vi "AbortSystemConfiguration.vi"(0 "File Path":path) -> ()   [LabVIEW 2021]
uses:
  <vilib>/Utility/file.llb/Write Delimited Spreadsheet (string).vi
  <vilib>/Utility/file.llb/Write Delimited Spreadsheet (I64).vi
  <vilib>/Utility/file.llb/Write Delimited Spreadsheet (DBL).vi
panel:
  in  "?":bool
  in  "?":bool
  out "Row":i32[](array[numeric])
  in  "Row":i32
  in  "Remove Event":bool
  in  "Add Event":bool
  in  "Sensor Select":u16(ring) items=["", "PT1", "PT2", "PT3", "TC1", "TC2", "LP1", "VS", "VLJ", "VR", "N2O Flowrate", "Ethanol Flowrate"]
  in  "Low Threshold":dbl
  in  "High Threshold":dbl
  in  "P#":i32
  in  "Event Name":string
  in  "SV6":bool
  in  "SV5":bool
  out "?":bool[](array[boolean])
  out "?":bool[](array[boolean])
  in  "SV4":bool
  out "?":bool[](array[boolean])
  in  "SV3":bool
  in  "SV2":bool
  in  "SV1":bool
  out "?":bool[](array[boolean])
  out "?":bool[](array[boolean])
  out "?":bool[](array[boolean])
  in  "SV0":bool
  out "?":dbl[](array[numeric])
  out "?":u16[](array[ring]) items=["", "PT1", "PT2", "PT3", "TC1", "TC2", "LP1", "VS", "VLJ", "VR", "N2O FLowrate", "Ethanol Flowrate"]
  out "?":string[](array[string])
  out "?":bool[](array[boolean])
  out "?":i32[](array[numeric])
  out "?":dbl[](array[numeric])
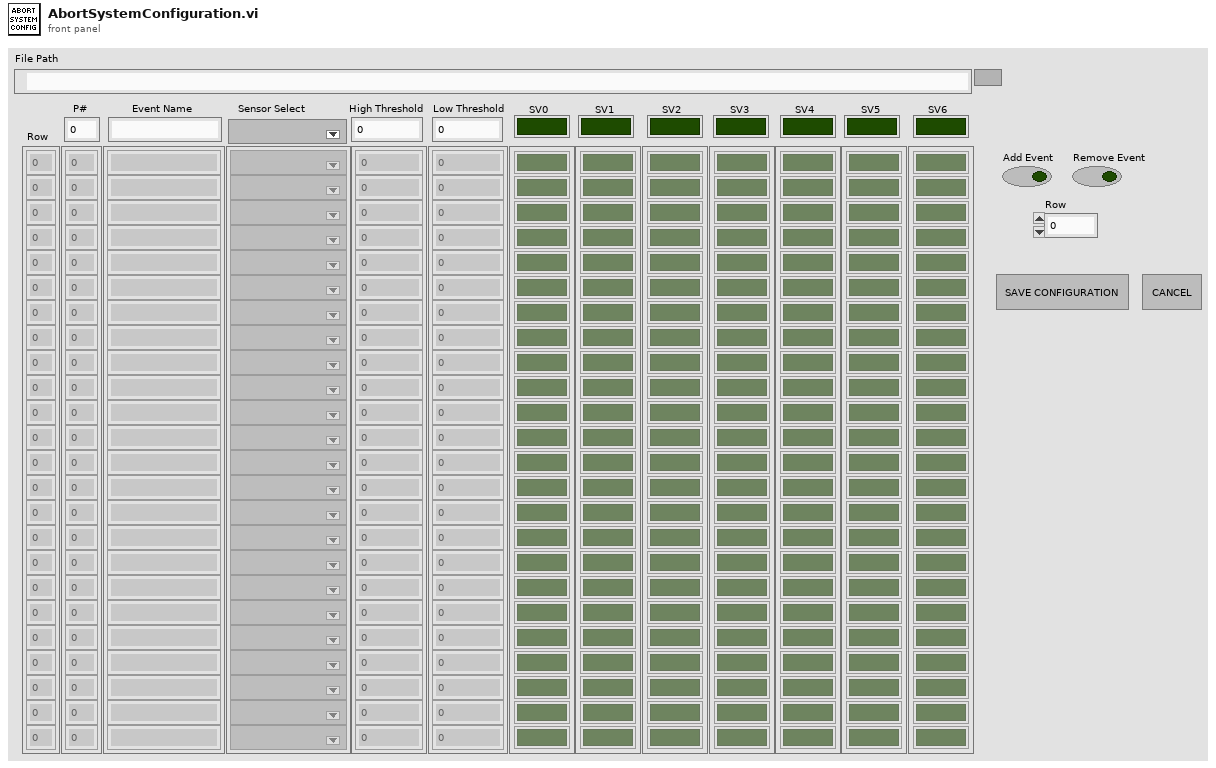
[diagram p1: front panel]
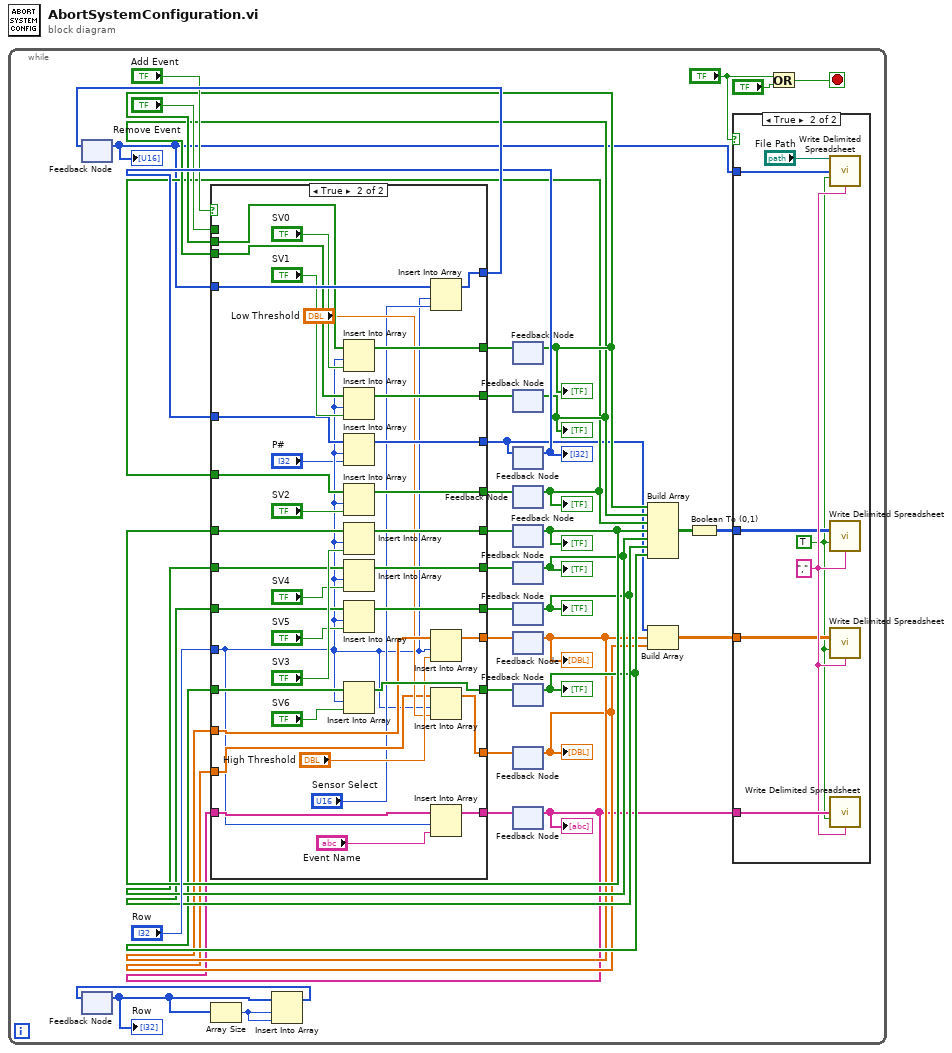
[diagram p0: block diagram]
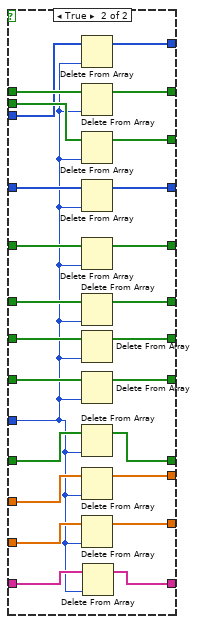
[diagram p4: hidden frame]
diagram:
  n1 = while {
    stop <- w3 stop-if-true
    n2 = feedback #1() -> (w5:u16[])  [unwired: 1 in]
    "?" <- w5
    n3 = feedback #2() -> (w22:i32[])  [unwired: 1 in]
    "Row" <- w22
    n4 = Array Size(array=w22) -> (size(s)=w21:i32)
    n5 = Insert Into Array(array=w22, index=w21, new element=w21) -> (w23:i32[])
    n6 = feedback-in #2(w23) -> ()
    n7 = feedback #3() -> (w18:bool[])  [unwired: 1 in]
    "?" <- w18
    n8 = feedback #4() -> (w17:bool[])  [unwired: 1 in]
    "?" <- w17
    n9 = feedback #5() -> (w27:i32[])  [unwired: 1 in]
    "?" <- w27
    n10 = feedback #6() -> (w16:bool[])  [unwired: 1 in]
    "?" <- w16
    n11 = feedback #7() -> (w15:bool[])  [unwired: 1 in]
    "?" <- w15
    n12 = feedback #8() -> (w14:bool[])  [unwired: 1 in]
    "?" <- w14
    n13 = feedback #9() -> (w13:bool[])  [unwired: 1 in]
    "?" <- w13
    n14 = feedback #10() -> (w11:dbl[])  [unwired: 1 in]
    "?" <- w11
    n15 = feedback #11() -> (w12:bool[])  [unwired: 1 in]
    "?" <- w12
    n16 = feedback #12() -> (w10:dbl[])  [unwired: 1 in]
    "?" <- w10
    n17 = feedback #13() -> (w8:string[])  [unwired: 1 in]
    "?" <- w8
    n18 = case shown="True" "Add Event" {
      tunnel: "Row" -> [w44 w108]
      tunnel: [w57 w143] -> w36
      tunnel: w5 -> [w56 w142]
      tunnel: [w63 w139] -> w35
      tunnel: w18 -> [w62 w138]
      tunnel: [w60 w137] -> w34
      tunnel: w17 -> [w61 w136]
      tunnel: [w69 w134] -> w33
      tunnel: w16 -> [w68 w133]
      tunnel: w15 -> [w66 w131]
      tunnel: [w67 w130] -> w32
      tunnel: w14 -> [w64 w128]
      tunnel: [w65 w127] -> w31
      tunnel: w13 -> [w58 w125]
      tunnel: [w59 w124] -> w30
      tunnel: w12 -> [w55 w123]
      tunnel: [w54 w122] -> w29
      tunnel: w8 -> [w52 w120]
      tunnel: [w53 w119] -> w28
      tunnel: w27 -> [w50 w117]
      tunnel: [w51 w116] -> w9
      tunnel: w11 -> [w46 w114]
      tunnel: [w47 w113] -> w26
      tunnel: w10 -> [w48 w111]
      tunnel: [w49 w110] -> w25
      tunnel: "Remove Event" -> [w45 _]
      frame False {
        n19 = case shown="False" w45 {
          tunnel: [w70 w106] -> w69
          tunnel: w68 -> [w70 w105]
          tunnel: [w72 w104] -> w67
          tunnel: w66 -> [w72 w103]
          tunnel: [w73 w102] -> w65
          tunnel: w64 -> [w73 w101]
          tunnel: [w74 w100] -> w63
          tunnel: w62 -> [w74 w99]
          tunnel: w61 -> [w76 w98]
          tunnel: [w76 w97] -> w60
          tunnel: [w77 w96] -> w59
          tunnel: w58 -> [w77 w95]
          tunnel: [w71 w94] -> w57
          tunnel: w56 -> [w71 w93]
          tunnel: w55 -> [w81 w92]
          tunnel: [w81 w91] -> w54
          tunnel: [w80 w90] -> w53
          tunnel: w52 -> [w80 w89]
          tunnel: [w79 w88] -> w51
          tunnel: w50 -> [w79 w87]
          tunnel: [w78 w86] -> w49
          tunnel: w48 -> [w78 w85]
          tunnel: [w75 w84] -> w47
          tunnel: w46 -> [w75 w83]
          tunnel: w44 -> [_ w82]
          frame False {
          }
          frame True {
            n20 = Delete From Array(array=w93, index=w82) -> (array with subset deleted=w94:u16[])  [unwired: 1 in, 1 out]
            n21 = Delete From Array(array=w99, index=w82) -> (array with subset deleted=w100:bool[])  [unwired: 1 in, 1 out]
            n22 = Delete From Array(array=w98, index=w82) -> (array with subset deleted=w97:bool[])  [unwired: 1 in, 1 out]
            n23 = Delete From Array(array=w87, index=w82) -> (array with subset deleted=w88:i32[])  [unwired: 1 in, 1 out]
            n24 = Delete From Array(array=w105, index=w82) -> (array with subset deleted=w106:bool[])  [unwired: 1 in, 1 out]
            n25 = Delete From Array(array=w103, index=w82) -> (array with subset deleted=w104:bool[])  [unwired: 1 in, 1 out]
            n26 = Delete From Array(array=w101, index=w82) -> (array with subset deleted=w102:bool[])  [unwired: 1 in, 1 out]
            n27 = Delete From Array(array=w95, index=w82) -> (array with subset deleted=w96:bool[])  [unwired: 1 in, 1 out]
            n28 = Delete From Array(array=w92, index=w82) -> (array with subset deleted=w91:bool[])  [unwired: 1 in, 1 out]
            n29 = Delete From Array(array=w83, index=w82) -> (array with subset deleted=w84:dbl[])  [unwired: 1 in, 1 out]
            n30 = Delete From Array(array=w85, index=w82) -> (array with subset deleted=w86:dbl[])  [unwired: 1 in, 1 out]
            n31 = Delete From Array(array=w89, index=w82) -> (array with subset deleted=w90:string[])  [unwired: 1 in, 1 out]
          }
        }
      }
      frame True {
        n32 = Insert Into Array(array=w138, index=w108, new element="SV0") -> (w139:bool[])
        n33 = Insert Into Array(array=w136, index=w108, new element="SV1") -> (w137:bool[])
        n34 = Insert Into Array(array=w117, index=w108, new element="P#") -> (w116:i32[])
        n35 = Insert Into Array(array=w133, index=w108, new element="SV2") -> (w134:bool[])
        n36 = Insert Into Array(array=w131, index=w108, new element="SV3") -> (w130:bool[])
        n37 = Insert Into Array(array=w128, index=w108, new element="SV4") -> (w127:bool[])
        n38 = Insert Into Array(array=w125, index=w108, new element="SV5") -> (w124:bool[])
        n39 = Insert Into Array(array=w123, index=w108, new element="SV6") -> (w122:bool[])
        n40 = Insert Into Array(array=w142, index=w108, new element="Sensor Select") -> (w143:u16[])
        n41 = Insert Into Array(array=w114, index=w108, new element="High Threshold") -> (w113:dbl[])
        n42 = Insert Into Array(array=w111, index=w108, new element="Low Threshold") -> (w110:dbl[])
        n43 = Insert Into Array(array=w120, index=w108, new element="Event Name") -> (w119:string[])
      }
    }
    n44 = feedback-in #1(w36) -> ()
    n45 = feedback-in #3(w35) -> ()
    n46 = feedback-in #4(w34) -> ()
    n47 = feedback-in #5(w9) -> ()
    n48 = feedback-in #6(w33) -> ()
    n49 = feedback-in #7(w32) -> ()
    n50 = feedback-in #8(w31) -> ()
    n51 = feedback-in #9(w30) -> ()
    n52 = feedback-in #10(w26) -> ()
    n53 = feedback-in #11(w29) -> ()
    n54 = feedback-in #12(w25) -> ()
    n55 = feedback-in #13(w28) -> ()
    n56 = Build Array(w18, w17, w16, w15, w14, w13, w12) -> (w7:bool[][])
    n57 = Build Array(w9, w11, w10) -> (w4:dbl[][])
    n58 = Boolean To (0,1)(Boolean=w7) -> (0, 1=w6:i16[][])
    n59 = case shown="True" "?" {
      tunnel: w6 -> [_ w41]
      tunnel: w4 -> [_ w39]
      tunnel: w5 -> [_ w40]
      tunnel: w8 -> [_ w43]
      frame False {
      }
      frame True {
        w38 = TRUE ("append to file? (new file:F)")
        w42 = "," ("delimiter (\\t)")
        n60 = call-poly <vilib>:"Write Delimited Spreadsheet.vi"("file path (dialog if empty)"="File Path", "1D data"=w40, "append to file? (new file:F)"=w38, "delimiter (\\t)"=w42) -> ()  [unwired: 10 in, 2 out]
        n61 = call-poly <vilib>:"Write Delimited Spreadsheet.vi"("2D data"=w41, "append to file? (new file:F)"=w38, "delimiter (\\t)"=w42) -> ()  [unwired: 11 in, 2 out]
        n62 = call-poly <vilib>:"Write Delimited Spreadsheet.vi"("2D data"=w39, "append to file? (new file:F)"=w38, "delimiter (\\t)"=w42) -> ()  [unwired: 11 in, 2 out]
        n63 = call-poly <vilib>:"Write Delimited Spreadsheet.vi"("1D data"=w43, "append to file? (new file:F)"=w38, "delimiter (\\t)"=w42) -> ()  [unwired: 11 in, 2 out]
      }
    }
    n64 = Or(x="?", y="?") -> (x .or. y?=w3:bool)
  }
